vi "niRFUtil WFM Histogram (DVR).vi"(0 "Data In":T3 min=0 max=127 format="%.2f", 1 "Histogram State Reference":T1, 5 "Max Bin":dbl format="%.2f", 7 "Min Bin":dbl format="%.2f", 9 "Bin Size":dbl format="%.2f", 11 "error in (no error)":errorcluster, 13 "Measurement Reset? (T)":T2=TRUE) -> (4 "Histogram Out":i32[](array[numeric]), 6 "Histogram Count":i32, 15 "error out":errorcluster)   [LabVIEW 2015, in "niRFUtil.lvlib"]
doc: "(c) Copyright 2006, National Instruments, Inc. This VI may not be duplicated, sold, or distributed without written consent from National Instruments."
uses:
  niRFUtil.lvlib
  Includes/niRFUtil INC Real Array.ctl
  Includes/niRFUtil INC Measurement Reset.ctl
  Includes/niRFUtil INC Histogram State Reference.ctl
  Includes/niRFUtil INC Histogram State Data.ctl
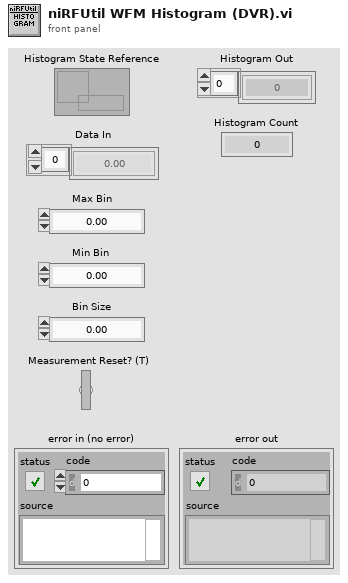
[diagram p1: front panel]
types:
  T1 = typedef "niRFUtil.lvlib/niRFUtil INC Histogram State Reference.ctl" = refnum<data-value>
  T2 = typedef "niRFUtil.lvlib/niRFUtil INC Measurement Reset.ctl" = bool
  T3 = typedef "niRFUtil.lvlib/niRFUtil INC Real Array.ctl" = sgl[]
  T4 = typedef "niRFUtil.lvlib/niRFUtil INC Histogram State Data.ctl" = cluster{"Accumulator":i32[], "Count":i32}
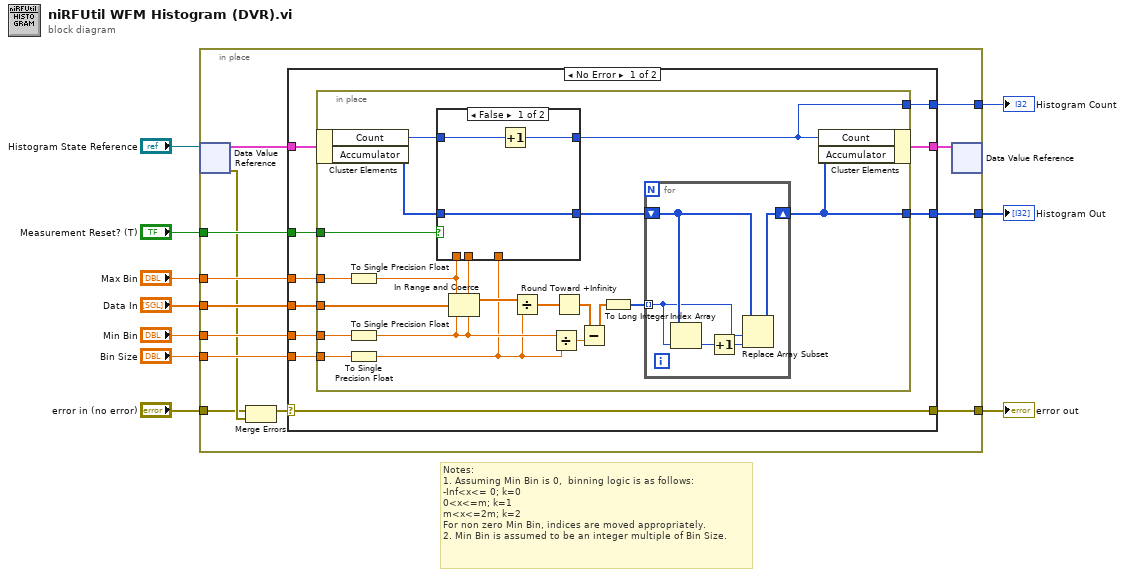
[diagram p0: block diagram]
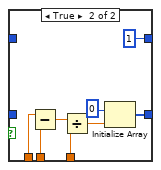
[diagram p2: hidden frame]
diagram:
  # "Notes: \n1. Assuming Min Bin is 0,  binning logic is as follows:\n-Inf<x<= 0; k=0\n0<x<=m; k=1\nm<x<=2m; k=2\nFor non zero Min Bin, indices are moved appropriately.\n2. Min Bin is assumed to be an integer multiple of Bin Size."
  n1 = in-place {
    in-place-border: "Data In" -> [w23]
    in-place-border: "Min Bin" -> [w22]
    in-place-border: "Max Bin" -> [w21]
    in-place-border: "Bin Size" -> [w20]
    in-place-border: [w19] -> w6
    in-place-border: "Measurement Reset? (T)" -> [w18]
    in-place-border: "error in (no error)" -> [w15]
    in-place-border: [w14] -> w2
    in-place-border: [w12] -> w1
    n2 = in-place-dvr #1("Histogram State Reference") -> (w13:T4, w17:errorcluster)
    n3 = Merge Errors(w15, w17) -> (w16:errorcluster)
    n4 = case shown="No Error" w16 {
      selector: w16 -> [w25 w70]
      tunnel: w23 -> [w33 _]
      tunnel: w22 -> [w32 _]
      tunnel: w21 -> [w31 _]
      tunnel: w20 -> [w30 _]
      tunnel: [w29 _] -> w19
      tunnel: w18 -> [w28 _]
      tunnel: [w25 w70] -> w14
      tunnel: w13 -> [w27 w69]
      tunnel: [w26 _] -> w12
      tunnel: [w24 w69] -> w11
      frame No Error {
        n5 = in-place {
          in-place-border: w33 -> [w34]
          in-place-border: w32 -> [w52]
          in-place-border: w31 -> [w51]
          in-place-border: w30 -> [w50]
          in-place-border: [w41] -> w29
          in-place-border: w28 -> [w49]
          in-place-border: [w39] -> w26
          n6 = in-place-cluster #2(w27) -> ("Count"=w40:i32, "Accumulator"=w42:i32[])
          n7 = To Single Precision Float(number=w51) -> (single precision float=w38:sgl)
          n8 = To Single Precision Float(number=w52) -> (single precision float=w37:sgl)
          n9 = To Single Precision Float(number=w50) -> (single precision float=w36:sgl)
          n10 = case shown="False" w49 {
            tunnel: w38 -> [_ w60]
            tunnel: w37 -> [_ w59]
            tunnel: w36 -> [_ w58]
            tunnel: [w55 w57] -> w43
            tunnel: w42 -> [w55 _]
            tunnel: [w53 1] -> w39
            tunnel: w40 -> [w54 _]
            frame False {
              n11 = Increment(x=w54) -> (x+1=w53:i32)
            }
            frame True {
              n12 = Subtract(x=w60, y=w59) -> (x-y=w62:sgl)
              n13 = Divide(x=w62, y=w58) -> (x/y=w61:sgl)
              n14 = Initialize Array(0 ("Numeric"), w61) -> (w57:i32[])
            }
          }
          n15 = In Range and Coerce(upper limit=w38, x=w34, lower limit=w37) -> (coerced(x)=w48:sgl[])  [unwired: 1 out]
          n16 = Divide(x=w48, y=w36) -> (x/y=w45:sgl[])
          n17 = Divide(x=w37, y=w36) -> (x/y=w46:sgl)
          n18 = Round Toward +Infinity(x=w45) -> (ceil(x): smallest int >= x=w35:sgl[])
          n19 = Subtract(x=w35, y=w46) -> (x-y=w44:sgl[])
          n20 = To Long Integer(number=w44) -> (32bit integer=w47:i32[])
          n21 = for {
            tunnel: w47 -> [w64] mode=indexing
            shift-right: [w65] -> w41
            shift-left: w43 -> [w66]
            n22 = Index Array(array=w66, index=w64) -> (element=w68:i32)
            n23 = Increment(x=w68) -> (x+1=w67:i32)
            n24 = Replace Array Subset(array=w66, new element=w67, index=w64) -> (w65:i32[])
          }
          n25 = in-place-cluster #2("Count"=w39, "Accumulator"=w41) -> (w24:T4)
        }
      }
      frame Error {
      }
    }
    n26 = in-place-dvr #1(w11) -> ()  [unwired: 2 out]
  }
  "Histogram Out" <- w6
  "error out" <- w2
  "Histogram Count" <- w1
